vi "BombedWallParamsStack.vi"(8 "error in (no error)":errorcluster, 11 "Bomb":bool) -> (0 "error out":errorcluster, 2 "HierarchyParams":variant[](array[variant]), 3 "BombedWall":refnum<class "BombedWall.lvclass">)   [LabVIEW 2020, in "BombedWall.lvclass"]
uses:
  BombedWall.lvclass
  Protected/property/Read BombedWallParams.vi
  BombedWall.lvclass/BombedWall.ctl
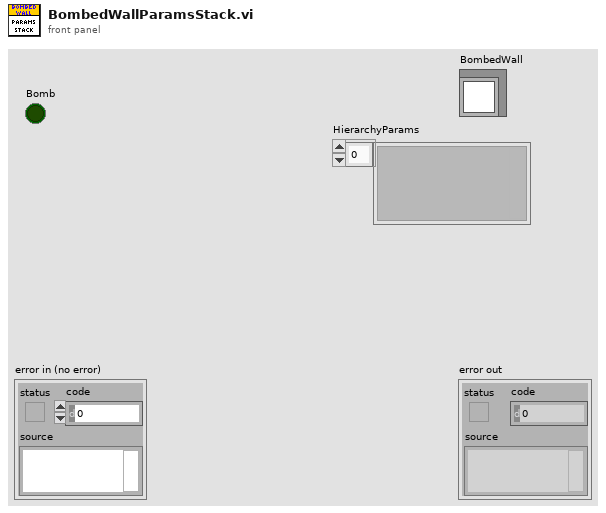
[diagram p1: front panel]
types:
  T1 = typedef "BombedWall.lvclass/BombedWallParams.ctl" = cluster{"bomb":bool}
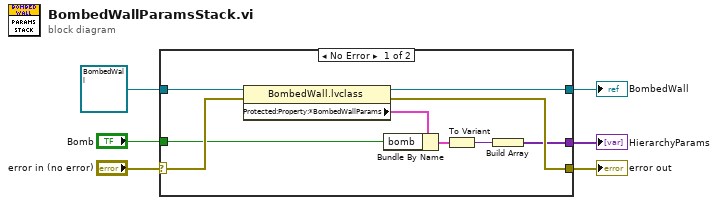
[diagram p0: block diagram]
diagram:
  n1 = case shown="No Error" "error in (no error)" {
    selector: "error in (no error)" -> [w15 w17]
    tunnel: [w12 w17] -> w5
    tunnel: "Bomb" -> [w11 _]
    tunnel: refnum<class "BombedWall.lvclass"> refnum ("Milk") -> [w14 w16]
    tunnel: [w13 w16] -> w3
    tunnel: [w10 _] -> w2
    frame No Error {
      n2 = property class="BombedWall.lvclass"(reference=w14, error in=w15) -> (reference out=w13:refnum<class "BombedWall.lvclass">, error out=w12:errorcluster, "Protected:Property:*BombedWallParams"=w7:T1)
      n3 = Bundle By Name(cluster=w7, "bomb"=w11) -> (w9:T1)
      n4 = To Variant(anything=w9) -> (Variant=w8:variant)
      n5 = Build Array(w8) -> (w10:variant[])
    }
    frame Error {
    }
  }
  "error out" <- w5
  "BombedWall" <- w3
  "HierarchyParams" <- w2
